vi "Init.vi"(3 "Container State":T6, 4 "Previous State":variant, 5 "Previous Version":T5) -> (2 "Current State":T1)   [LabVIEW 2015, in "SignalManager.xctl"]
uses:
  SignalManager.xctl
  State.ctl
  Utility VIs/Controls/KListboxEx/Events.ctl
  Utility VIs/Controls/KListboxEx/Event Action.ctl
  PeriodDisplay.ctl
  Events.ctl
  Event Data.ctl
  <vilib>/_xctls/Container State.ctl
  <vilib>/_xctls/Version.ctl
  Utility VIs/Controls/KListboxEx/KListboxEx.xctl
  <vilib>/_xctls/XControlSupport.lvlib
panel:
  in  "Default Indicator State":T1
  in  "Default Control State":T1
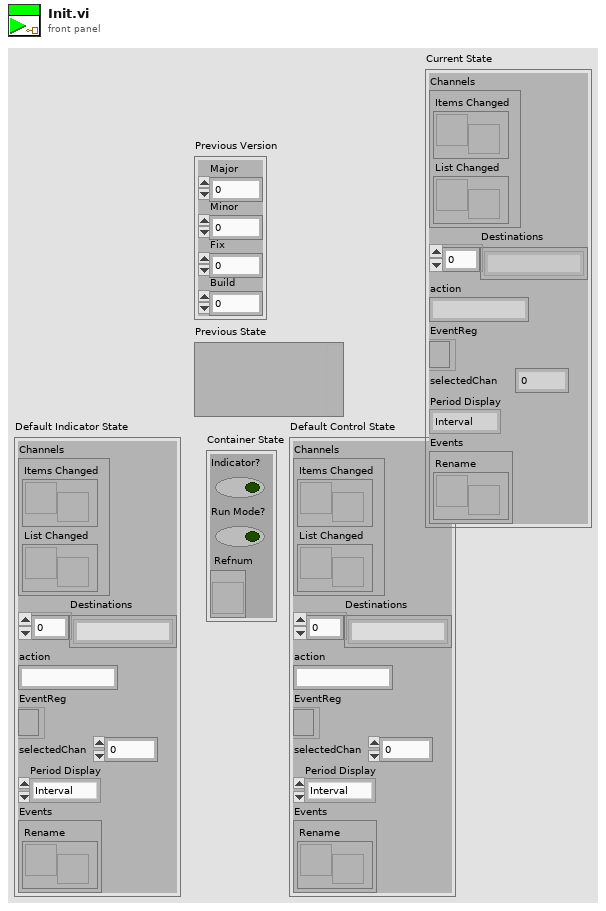
[diagram p1: front panel]
types:
  T1 = typedef "SignalManager.xctl/State.ctl" = cluster{"Channels":T2, "Destinations":string[], "action":string, "EventReg":refnum<event-registration>, "selectedChan":i32, "Period Display":T3, "Events":T4}
  T2 = typedef "KListboxEx.xctl/Events.ctl" = cluster{"Items Changed":refnum<user-event>, "List Changed":refnum<user-event>}
  T3 = typedef "SignalManager.xctl/PeriodDisplay.ctl" = enum16{"Interval", "RepRate", "Both"}
  T4 = typedef "SignalManager.xctl/Events.ctl" = cluster{"Rename":refnum<user-event>}
  T5 = typedef "XControlSupport.lvlib/Version.ctl" = cluster{"Major":u16, "Minor":u16, "Fix":u16, "Build":u16}
  T6 = typedef "XControlSupport.lvlib/Container State.ctl" = cluster{"Indicator?":bool, "Run Mode?":bool, " Refnum":refnum<vi>}
  T7 = typedef "KListboxEx.xctl/Event Action.ctl" = enum16{"None", "Add", "Delete", "Move", "Edit", "Select"}
  T8 = cluster{"Action":T7, "Name":string, "Start row":i32, "End row":i32}
  T9 = cluster{"Data":refnum<user-event>, "Data":refnum<user-event>}
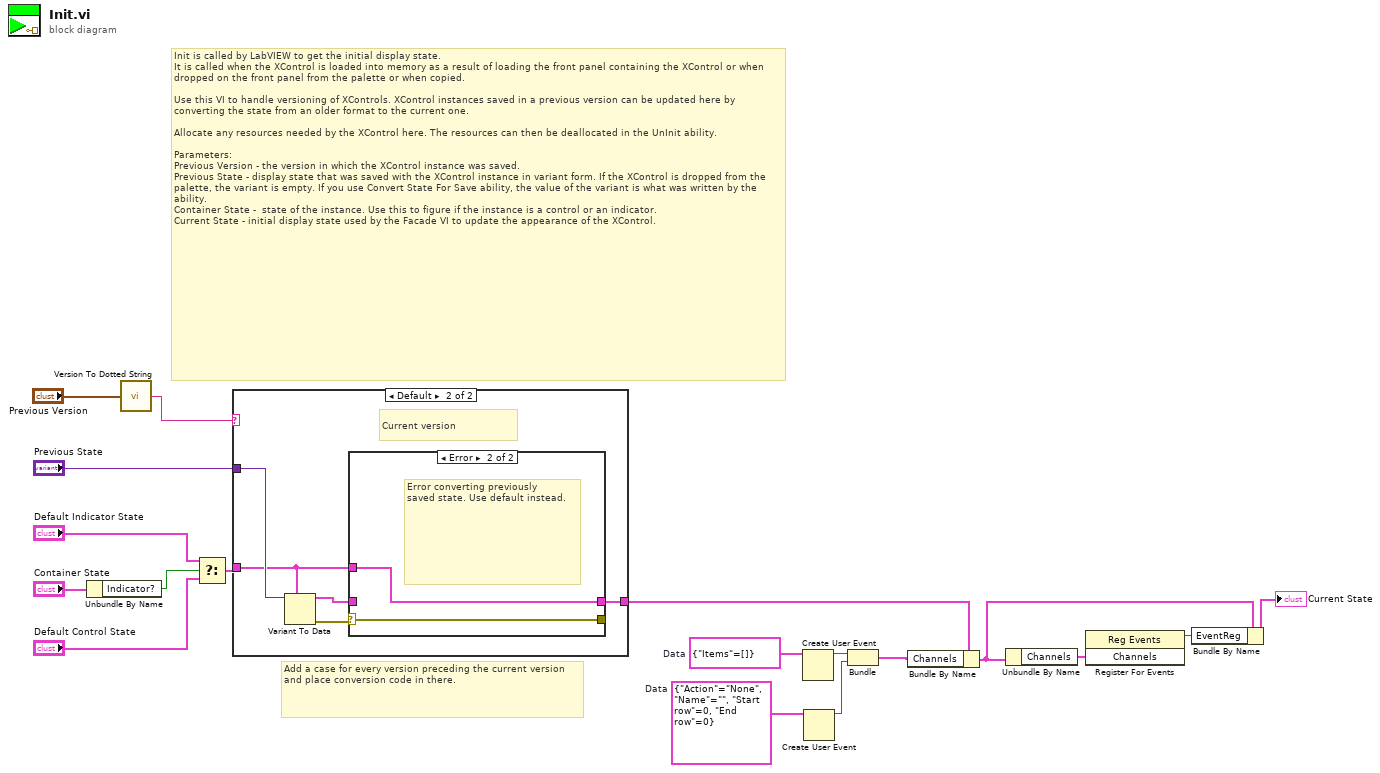
[diagram p0: block diagram]
diagram:
  w7 = T8 {"Action"=enum."None", "Name"="", "Start row"=0, "End row"=0}  # Data
  w9 = cluster{"Items":string[]} {"Items"=[]}  # Data
  # "Add a case for every version preceding the current version and place conversion code in there."
  # "Init is called by LabVIEW to get the initial display state.\nIt is called when the XControl is loaded into memory as a result of loading the front panel containing the XControl or when dropped on the front panel from the palette or when copied.\n\nUse this VI to handle versioning of XControls. XControl instances saved in a previous version can be updated here by converting the state from an older format to the current one.\n\nAllocate any resources needed by the XControl here. The resources can then be deallocated in the UnInit ability.\n\nParameters:\nPrevious Version - the version in which the XControl instance was saved.\nPrevious State - display state that was saved with the XControl instance in variant form. If the XControl is dropped from the palette, the variant is empty. If you use Convert State For Save ability, the value of the variant is what was written by the ability. \nContainer State -  state of the instance. Use this to figure if the instance is a control or an indicator.\nCurrent State - initial display state used by the Facade VI to update the appearance of the XControl."
  n1 = Unbundle By Name("Container State") -> ("Indicator?"=w13:bool)
  n2 = call <vilib>:"Version To Dotted String.vi"("Version"="Previous Version") -> ("String Version"=w10:string)
  n3 = Select(t="Default Indicator State", s=w13, f="Default Control State") -> (s? t:f=w12:T1)
  n4 = case shown="Default" w10 {
    tunnel: "Previous State" -> [_ w24]
    tunnel: [w19 w20] -> w17
    tunnel: w12 -> [w19 w21]
    frame "0.0.0.0" {
      # "Just created, use default state"
    }
    frame Default {
      # "Current version"
      n5 = Variant To Data(type=w21, Variant=w24) -> (data=w22:T1, error out=w23:errorcluster)  [unwired: 1 in]
      n6 = case shown="Error" w23 {
        selector: w23 -> [w26 w27]
        tunnel: w22 -> [w25 _]
        tunnel: [w25 w28] -> w20
        tunnel: w21 -> [_ w28]
        tunnel: [w26 w27] -> _
        frame No Error {
        }
        frame Error {
          # "Error converting previously \nsaved state. Use default instead."
        }
      }
    }
  }
  n7 = Create User Event(user event datatype=w9) -> (user event=w8:refnum<user-event>)  [unwired: 1 in, 1 out]
  n8 = Create User Event(user event datatype=w7) -> (user event=w6:refnum<user-event>)  [unwired: 1 in, 1 out]
  n9 = Bundle("Data"=w8, "Data"=w6) -> (w5:T9)  [unwired: 1 in]
  n10 = Bundle By Name(cluster=w17, "Channels"=w5) -> (w4:T1)
  n11 = Unbundle By Name(w4) -> ("Channels"=w2:T2)
  n12 = register-events(w2) -> (reference out=w1:refnum<event-registration>)  [unwired: 2 in, 1 out]
  n13 = Bundle By Name(cluster=w4, "EventReg"=w1) -> (→"Current State":T1)
